vi "$TXXX.vi"(11 "反馈信息":string) -> (3 "接收信息":T1 {"校验和" format="%01xH"; "信息内容"."CRC标志" format="%01xH"; "信息内容"."发信时间分" format="%0d"; "信息内容"."发信时间时" format="%0d"; "信息内容"."发信方地址" format="%0d"; "信息内容"."信息类别" format="%01xH"})   [LabVIEW 2016, in "环境动力监测库.lvlib" / "NMEA.lvlib"]
uses:
  NMEA.lvlib
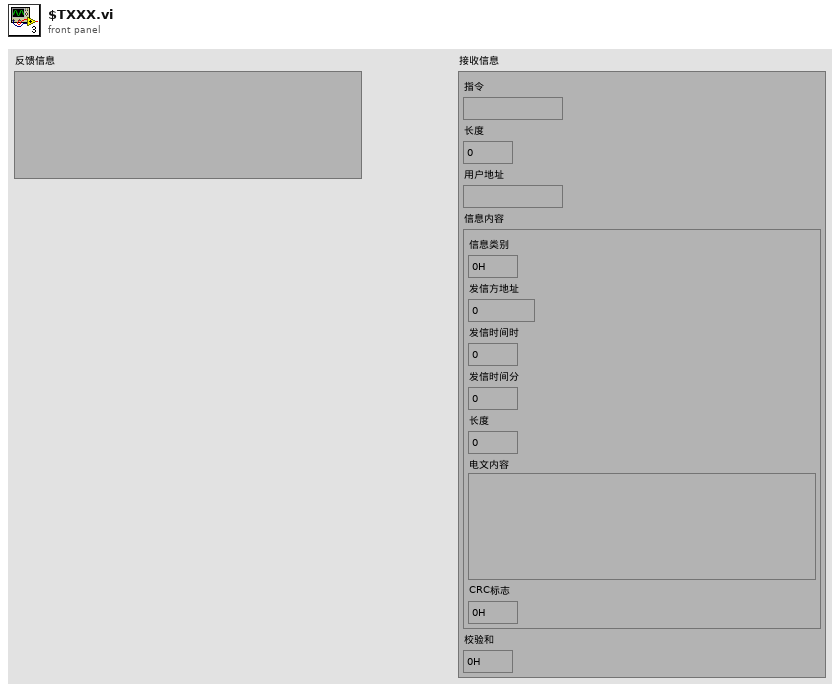
[diagram p1: front panel]
types:
  T1 = cluster{"指令":string, "长度":u16, "用户地址":string, "信息内容":cluster{"信息类别":u8, "发信方地址":u32, "发信时间时":u8, "发信时间分":u8, "长度":u16, "电文内容":string, "CRC标志":u8}, "校验和":u8}
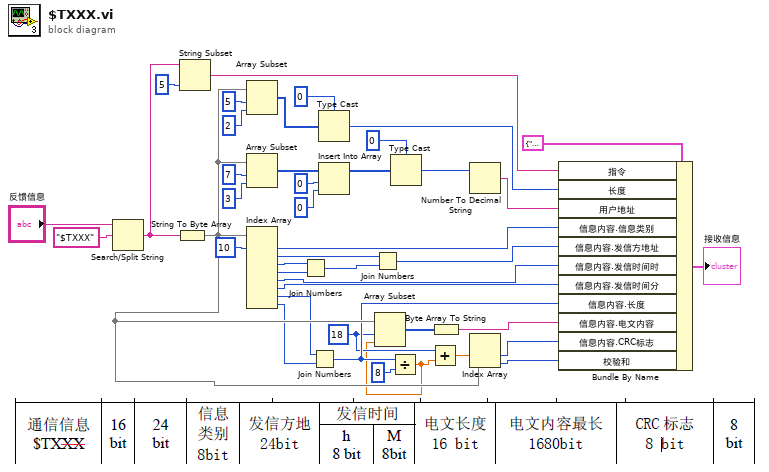
[diagram p0: block diagram]
diagram:
  w9 = 18 ("索引")
  n1 = Search/Split String(string="反馈信息", search string/char (-)="$TXXX" ("搜索字符串/字符(-)")) -> (match + rest of string=w38:string)  [unwired: 1 in, 2 out]
  n2 = String To Byte Array(string=w38) -> (unsigned byte array=w12:u8[])
  n3 = String Subset(string=w38, length (rest)=5 ("长度（剩余）")) -> (substring=w37:string)  [unwired: 1 in]
  n4 = Array Subset(array=w12, index=5 ("索引"), length=2 ("长度")) -> (w34:u8[])
  n5 = Array Subset(array=w12, index=7 ("索引"), length=3 ("长度")) -> (w29:u8[])
  n6 = Index Array(array=w12, index #1=10 ("索引")) -> (element #1=w22:u8, element #2=w16:u8, element #3=w18:u8, element #4=w19:u8, element #5=w1:u8, element #6=w2:u8, element #7=w3:u8, element #8=w4:u8)  [unwired: 7 in]
  n7 = Join Numbers(hi=w18, lo=w19) -> ((hi.lo)=w17:u16)
  n8 = Join Numbers(hi=w3, lo=w4) -> ((hi.lo)=w10:u16)
  n9 = Type Cast(type=u16 0 ("长度"), x=w34) -> (*(type *) &x=w32:u16)
  n10 = Insert Into Array(array=w29, index=0 ("索引"), new element=u8 0 ("新元素/子数组")) -> (w26:u8[])
  n11 = Join Numbers(hi=w16, lo=w17) -> ((hi.lo)=w15:u32)
  n12 = Divide(x=w10, y=u16 8) -> (x/y=w5:dbl)
  n13 = Array Subset(array=w12, index=w9, length=w5) -> (w14:u8[])
  n14 = Type Cast(type=u32 0 ("长度"), x=w26) -> (*(type *) &x=w27:u32)
  n15 = Add(x=w9, y=w5) -> (x+y=w11:dbl)
  n16 = Byte Array To String(unsigned byte array=w14) -> (string=w13:string)
  n17 = Number To Decimal String(number=w27) -> (decimal integer string=w23:string)  [unwired: 1 in]
  n18 = Index Array(array=w12, index #1=w11) -> (element #1=w8:u8, element #2=w7:u8)  [unwired: 1 in]
  n19 = Bundle By Name(cluster=T1 {"指令"="", "长度"=0, "用户地址"="", "信息内容"={"信息类别"=0, "发信方地址"=0, "发信时间时"=0, "发信时间分"=0, "长度"=0, "电文内容"="", "CRC标志"=0}, "校验和"=0} ("接收信息"), "指令"=w37, "长度"=w32, "用户地址"=w23, "信息内容.信息类别"=w22, "信息内容.发信方地址"=w15, "信息内容.发信时间时"=w1, "信息内容.发信时间分"=w2, "信息内容.长度"=w10, "信息内容.电文内容"=w13, "信息内容.CRC标志"=w8, "校验和"=w7) -> (→"接收信息":T1)
